vi "AlliGator Compute ROI Decay.vi"(5 "Pixel Threshold High":dbl, 6 "Loop ID":i32, 7 "Pixel Threshold Low":dbl, 8 "error in (no error)":errorcluster, 9 "Decay Peak  Constraints":T2, 10 "ROI Descriptor":T1 {"Contours"."Type" items=["No Selection", "Point", "Line", "Rectangle", "Oval", "Polygon", "Freehand Region", "Annulus", "Unused2", "Unused3", "Broken Line", "Freehand Line", "Rotated Rectangle"]}, 11 "Images":cluster{"Image Sum":T3, "Image Array":T3[]}) -> (0 "error out":errorcluster, 1 "# Valid Pixels":i32, 2 "ROI Center":cluster{"X":i32, "Y":i32}, 3 "Decay Points":dbl[](array[numeric]), 4 "# Pixels":i32)   [LabVIEW 2021, in "AlliGator Decay Processing.lvlib"]
doc: "Extracts the ROI pixel intensities for the different gate images, rejecting pixels not satisfying the intensity-based or peak-intensity based criteria.\n\nA different (faster) approach is used for single-pixel ROIs."
uses:
  AlliGator Decay Processing.lvlib
  <vilib>/vision/Image Controls.llb/IMAQ Image.ctl
  Comparison/Is Valid Number (SGL Array).vi
  Arrays/Replace NaN by 0 (2D SGL).vi/df975b44-f6c5-4554-af30-980613d33749.vi
  Comparison/Is a Valid Number (SGL).vi
  <vilib>/Utility/error.llb/Error Cluster From Error Code.vi
  <vilib>/vision/EDVR.llb/IMAQ ImageToEDVR 2D U8.vi
  <vilib>/vision/EDVR.llb/IMAQ ImageToEDVR 2D I16.vi
  <vilib>/vision/EDVR.llb/IMAQ ImageToEDVR 2D SGL.vi
  <vilib>/vision/EDVR.llb/IMAQ ImageToEDVR 2D U16.vi
  <vilib>/ErrorRing/Error Ring.xnode
  Source Image/AlliGator Source Image.lvlib
  <vilib>/vision/NI_Vision_Development_Module.lvlib
  Arrays/Arrays.lvlib
  Image/Image.lvlib
  Comparison/Comparison.lvlib
  Error/Error.lvlib
  Time/Time.lvlib
panel:
  out "CPU (s)":dbl
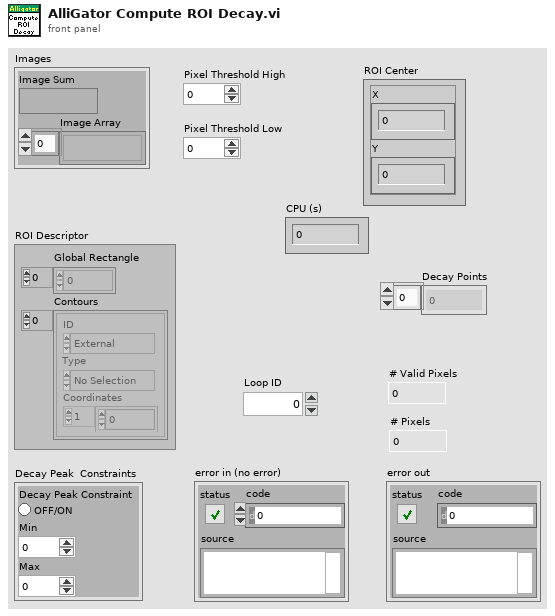
[diagram p1: front panel]
types:
  T1 = typedef "ROI Descriptor" = cluster{"Global Rectangle":i32[], "Contours":cluster{"ID":enum32{"External", "Internal"}, "Type":u32, "Coordinates":i32[]}[]}
  T2 = cluster{"Decay Peak Constraint":bool, "Min":dbl, "Max":dbl}
  T3 = typedef "IMAQ Image.ctl" = refnum<image>
  T4 = typedef "IMAQ Point" = cluster{"X":sgl, "Y":sgl}
  T5 = typedef "Image Type" = u32
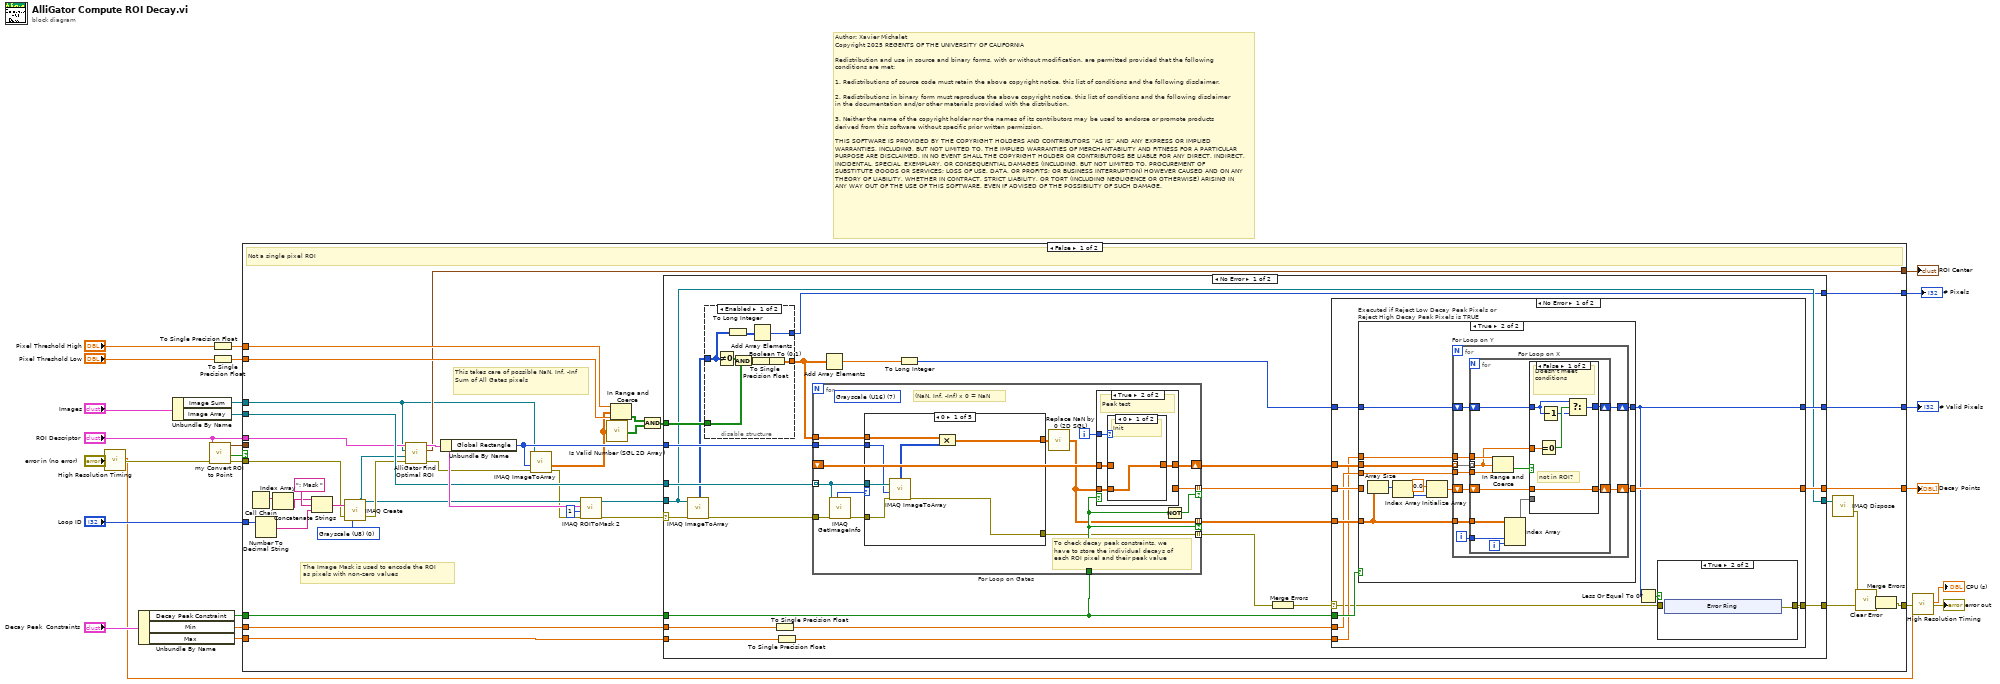
[diagram p0: block diagram]
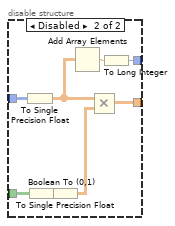
[diagram p2: hidden frame]
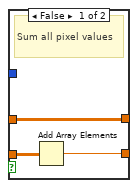
[diagram p3: hidden frame]
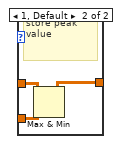
[diagram p4: hidden frame]
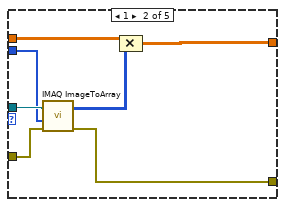
[diagram p5: hidden frame]
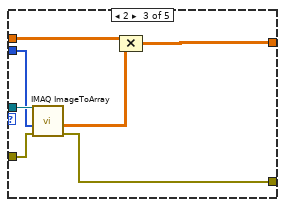
[diagram p6: hidden frame]
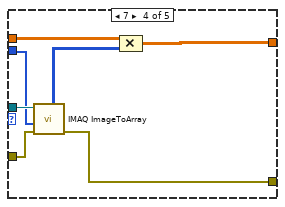
[diagram p7: hidden frame]
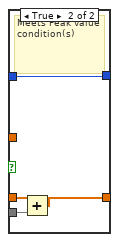
[diagram p11: hidden frame]
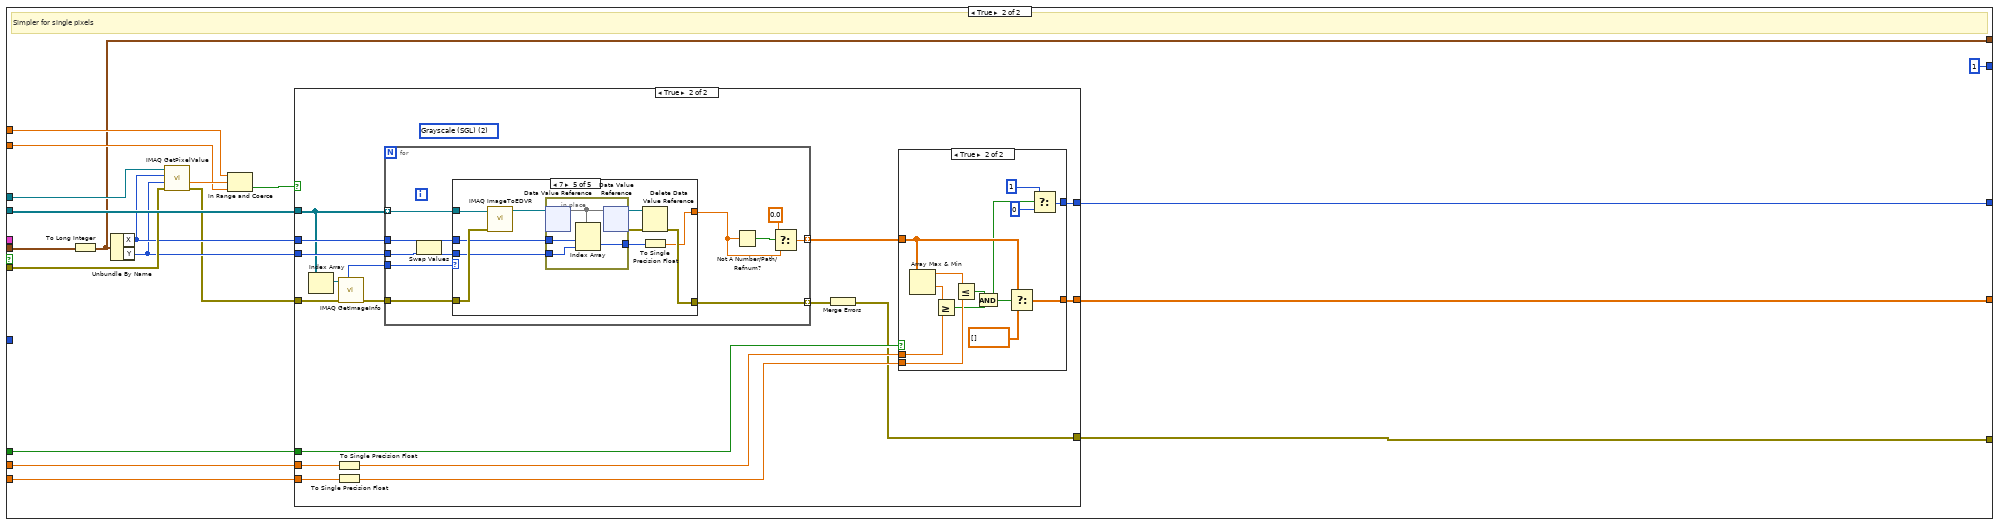
[diagram p14: hidden frame]
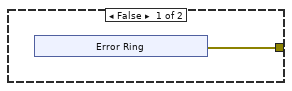
[diagram p15: hidden frame]
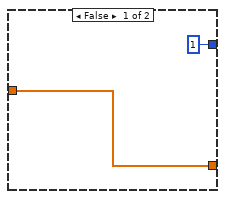
[diagram p16: hidden frame]
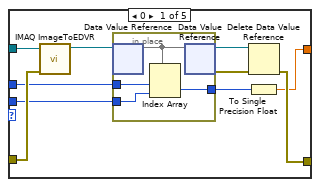
[diagram p17: hidden frame]
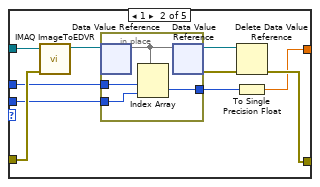
[diagram p18: hidden frame]
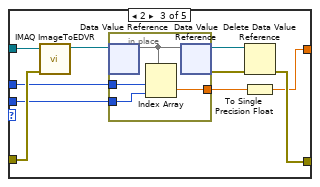
[diagram p19: hidden frame]
diagram:
  # "Author: Xavier Michalet\nCopyright 2025 REGENTS OF THE UNIVERSITY OF CALIFORNIA\n\nRedistribution and use in source and binary forms, with or without modification, are permitted provided that the following conditions are met:\n\n1. Redistributions of source code must retain the above copyright notice, this list of conditions and the following disclaimer.\n\n2. Redistributions in binary form must reproduce the above copyright notice, this list of conditions and the following disclaimer in the documentation and/or other materials provided with the distribution.\n\n3. Neither the name of the copyright holder nor the names of its contributors may be used to endorse or promote products derived from this software without specific prior written permission.\n\nTHIS SOFTWARE IS PROVIDED BY THE COPYRIGHT HOLDERS AND CONTRIBUTORS “AS IS” AND ANY EXPRESS OR IMPLIED WARRANTIES, INCLUDING, BUT NOT LIMITED TO, THE IMPLIED WARRANTIES OF MERCHANTABILITY AND FITNESS FOR A PARTICULAR PURPOSE ARE DISCLAIMED. IN NO EVENT SHALL THE COPYRIGHT HOLDER OR CONTRIBUTORS BE LIABLE FOR ANY DIRECT, INDIRECT, INCIDENTAL, SPECIAL, EXEMPLARY, OR CONSEQUENTIAL DAMAGES (INCLUDING, BUT NOT LIMITED TO, PROCUREMENT OF SUBSTITUTE GOODS OR SERVICES; LOSS OF USE, DATA, OR PROFITS; OR BUSINESS INTERRUPTION) HOWEVER CAUSED AND ON ANY THEORY OF LIABILITY, WHETHER IN CONTRACT, STRICT LIABILITY, OR TORT (INCLUDING NEGLIGENCE OR OTHERWISE) ARISING IN ANY WAY OUT OF THE USE OF THIS SOFTWARE, EVEN IF ADVISED OF THE POSSIBILITY OF SUCH DAMAGE."
  n1 = call "High Resolution Timing.vi"("Error In"="error in (no error)") -> ("elapsed (relative) seconds"=w1:dbl, "Error Out"=w4:errorcluster)  [unwired: 16 in, 1 out]
  n2 = Unbundle By Name("Decay Peak  Constraints") -> ("Decay Peak Constraint"=w23:bool, "Min"=w24:dbl, "Max"=w25:dbl)
  n3 = Unbundle By Name("Images") -> ("Image Sum"=w21:T3, "Image Array"=w13:T3[])
  n4 = call "my Convert ROI to Point.vi"("error in (no error)"=w4, "ROI Descriptor"="ROI Descriptor") -> ("error out"=w9:errorcluster, "Is a Point?"=w8:bool, "Point"=w6:T4)  [unwired: 6 in]
  n5 = To Single Precision Float(number="Pixel Threshold High") -> (single precision float=w19:sgl)
  n6 = To Single Precision Float(number="Pixel Threshold Low") -> (single precision float=w16:sgl)
  n7 = case shown="False" w8 {
    tunnel: w25 -> [w64 w232]
    tunnel: w24 -> [w63 w231]
    tunnel: w23 -> [w62 w233]
    tunnel: w21 -> [w30 w242]
    tunnel: [w29 w226] -> w20
    tunnel: w19 -> [w60 w239]
    tunnel: [w59 1] -> w17
    tunnel: w16 -> [w57 w238]
    tunnel: [w53 w227] -> w15
    tunnel: [w52 w230] -> w14
    tunnel: w13 -> [w51 w243]
    tunnel: [w50 w228] -> w12
    tunnel: w9 -> [w45 w241]
    tunnel: "ROI Descriptor" -> [w48 _]
    tunnel: w6 -> [_ w229]
    tunnel: "Loop ID" -> [w38 _]
    frame False {
      w41 = T5 0 items=["Grayscale (U8)", "Grayscale (I16)", "Grayscale (SGL)", "Complex (CSG)", "RGB (U32)", "HSL (U32)", "RGB (U64)", "Grayscale (U16)"] ("Image Type")
      # "This takes care of possible NaN, Inf, -Inf Sum of All Gates pixels"
      # "The Image Mask is used to encode the ROI\nas pixels with non-zero values"
      # "Not a single pixel ROI"
      n8 = Call Chain() -> (call chain=w39:string[])
      n9 = Number To Decimal String(number=w38) -> (decimal integer string=w37:string)  [unwired: 1 in]
      n10 = Index Array(array=w39) -> (element=w40:string)  [unwired: 1 in]
      n11 = Concatenate Strings(w40, ": Mask " ("string"), w37) -> (w47:string)
      n12 = call "IMAQ Create"("Image Name"=w47, "Image Type"=w41, "error in (no error)"=w45) -> ("New Image"=w42:T3, "error out"=w44:errorcluster)  [unwired: 2 in]
      n13 = call "AlliGator Find Optimal ROI.vi"("error in (no error)"=w44, "ROI Mask"=w42, "Image Sum"=w30, "ROI Descriptor in"=w48) -> ("error out"=w36:errorcluster, "ROI Center"=w50:cluster{"X":i32, "Y":i32}, "ROI Descriptor out"=w55:T1)  [unwired: 5 in]
      n14 = Unbundle By Name(w55) -> ("Global Rectangle"=w35:i32[])
      n15 = call "IMAQ ImageToArray"("error in (no error)"=w36, "Optional Rectangle"=w35, "Image"=w30) -> ("Image Pixels (Float)"=w34:sgl[][], "error out"=w31:errorcluster)  [unwired: 1 in, 3 out]
      n16 = call "IMAQ ROIToMask 2"("error in (no error)"=w31, "Filling Value (255)"=1, "ROI Descriptor"=w55, "Image"=w42) -> ("error out"=w49:errorcluster, "Image Out"=w54:T3)  [unwired: 5 in, 1 out]
      n17 = call "Is Valid Number (SGL 2D Array).vi"("SGL 2D Array"=w34) -> ("Is Valid Number? (2D)"=w32:bool[][])  [unwired: 8 in]
      n18 = In Range and Coerce(upper limit=w60, x=w34, lower limit=w57) -> (In Range?=w33:bool[][])  [unwired: 1 out]
      n19 = Compound Arithmetic op=AND(w33, w32) -> (w58:bool[][])
      n20 = case shown="No Error" w49 {
        selector: w49 -> [w74 w224]
        tunnel: w64 -> [w88 _]
        tunnel: w63 -> [w87 _]
        tunnel: w62 -> [w86 _]
        tunnel: [w71 w224] -> w61
        tunnel: [w65 _] -> w59
        tunnel: w58 -> [w84 _]
        tunnel: w35 -> [w83 _]
        tunnel: w54 -> [w72 w223]
        tunnel: [w81 _] -> w53
        tunnel: [w80 _] -> w52
        tunnel: w51 -> [w77 _]
        tunnel: [w72 w223] -> w43
        frame No Error {
          n21 = call "IMAQ ImageToArray"("error in (no error)"=w74, "Image"=w72) -> ("error out"=w67:errorcluster, "Image Pixels (U8)"=w69:u8[][])  [unwired: 2 in, 3 out]
          n22 = disable-structure shown="Enabled" {
            disable-tunnel: w84 -> [w96 w104]
            disable-tunnel: w69 -> [w91 w102]
            disable-tunnel: [w92 w98] -> w68
            disable-tunnel: [w89 w97] -> w65
            frame Enabled {
              n23 = Not Equal To 0?(x=w91) -> (x != 0?=w95:bool[][])
              n24 = To Long Integer(number=w91) -> (32bit integer=w90:i32[][])
              n25 = And(x=w96, y=w95) -> (x .and. y?=w94:bool[][])
              n26 = Boolean To (0,1)(Boolean=w94) -> (0, 1=w93:i16[][])
              n27 = Add Array Elements(numeric array=w90) -> (sum=w89:i32)
              n28 = To Single Precision Float(number=w93) -> (single precision float=w92:sgl[][])
            }
            frame Disabled {
              n29 = To Single Precision Float(number=w102) -> (single precision float=w100:sgl[][])
              n30 = Boolean To (0,1)(Boolean=w104) -> (0, 1=w103:i16[][])
              n31 = To Single Precision Float(number=w103) -> (single precision float=w99:sgl[][])
              n32 = Add Array Elements(numeric array=w100) -> (sum=w101:sgl)
              n33 = Multiply(x=w100, y=w99) -> (x*y=w98:sgl[][])
              n34 = To Long Integer(number=w101) -> (32bit integer=w97:i32)
            }
          }
          n35 = To Single Precision Float(number=w87) -> (single precision float=w76:sgl)
          n36 = To Single Precision Float(number=w88) -> (single precision float=w75:sgl)
          n37 = for "For Loop on Gates" {
            tunnel: w77 -> [w111] mode=indexing
            tunnel: [w117] -> w79 mode=indexing if=w115
            shift-right: [w119] -> w82
            shift-left: _ -> [w118]
            tunnel: w86 -> [w116]
            tunnel: [w105] -> w78 mode=indexing if=w116
            tunnel: w83 -> [w114]
            tunnel: w68 -> [w112]
            tunnel: [w109] -> w70 mode=indexing
            tunnel: w67 -> [w108]
            i -> [w113]
            (unwired) T5 7 items=["Grayscale (U8)", "Grayscale (I16)", "Grayscale (SGL)", "Complex (CSG)", "RGB (U32)", "HSL (U32)", "RGB (U64)", "Grayscale (U16)"] ("Image Type")
            # "(NaN, Inf, -Inf) x 0 = NaN"
            # "To check decay peak constraints, we have to store the individual decays of each ROI pixel and their peak value"
            n38 = call "IMAQ GetImageInfo"("error in (no error)"=w108, "Image"=w111) -> ("error out"=w106:errorcluster, "Image Type"=w110:T5)  [unwired: 2 in, 6 out]
            n39 = case shown="0" w110 {
              tunnel: [w137 w144 w151 w158 _] -> w107
              tunnel: w114 -> [w132 w138 w145 w152 _]
              tunnel: w112 -> [w136 w143 w150 w157 _]
              tunnel: w111 -> [w135 w142 w149 w156 _]
              tunnel: [w131 w140 w147 w154 w159] -> w109
              tunnel: w106 -> [w134 w141 w148 w155 w159]
              frame 0 {
                n40 = call "IMAQ ImageToArray"("error in (no error)"=w134, "Optional Rectangle"=w132, "Image"=w135) -> ("error out"=w131:errorcluster, "Image Pixels (U8)"=w133:u8[][])  [unwired: 1 in, 3 out]
                n41 = Compound Arithmetic op=MULTIPLY(w136, w133) -> (w137:sgl[][])
              }
              frame 1 {
                n42 = call "IMAQ ImageToArray"("error in (no error)"=w141, "Optional Rectangle"=w138, "Image"=w142) -> ("error out"=w140:errorcluster, "Image Pixels (I16)"=w139:i16[][])  [unwired: 1 in, 3 out]
                n43 = Compound Arithmetic op=MULTIPLY(w143, w139) -> (w144:sgl[][])
              }
              frame 2 {
                n44 = call "IMAQ ImageToArray"("error in (no error)"=w148, "Optional Rectangle"=w145, "Image"=w149) -> ("Image Pixels (Float)"=w146:sgl[][], "error out"=w147:errorcluster)  [unwired: 1 in, 3 out]
                n45 = Compound Arithmetic op=MULTIPLY(w150, w146) -> (w151:sgl[][])
              }
              frame 7 {
                n46 = call "IMAQ ImageToArray"("error in (no error)"=w155, "Optional Rectangle"=w152, "Image"=w156) -> ("Image Pixels (U16)"=w153:u16[][], "error out"=w154:errorcluster)  [unwired: 1 in, 3 out]
                n47 = Compound Arithmetic op=MULTIPLY(w157, w153) -> (w158:sgl[][])
              }
              frame 3, Default {
              }
            }
            n48 = call "Replace NaN by 0 (2D SGL).vi"("Array in"=w107) -> ("Array out"=w105:sgl[][])  [unwired: 8 in]
            n49 = case shown="True" w116 {
              tunnel: w113 -> [_ w126]
              tunnel: w105 -> [w121 w125]
              tunnel: [w122 w124] -> w119
              tunnel: w118 -> [w122 w123]
              tunnel: [w120 _] -> w117
              frame False {
                # "Sum all pixel values"
                n50 = Add Array Elements(numeric array=w121) -> (sum=w120:sgl)
              }
              frame True {
                # "Peak test"
                n51 = case shown="0" w126 {
                  tunnel: w125 -> [w127 w129]
                  tunnel: [w127 w128] -> w124
                  tunnel: w123 -> [_ w130]
                  frame 0 {
                    # "Init"
                  }
                  frame 1, Default {
                    # "store peak value"
                    n52 = Max & Min(x=w130, y=w129) -> (max(x,y)=w128:sgl[][])  [unwired: 1 out]
                  }
                }
              }
            }
            n53 = Not(x=w116) -> (.not. x?=w115:bool)
          }
          n54 = Add Array Elements(numeric array=w68) -> (sum=w85:sgl)
          n55 = To Long Integer(number=w85) -> (32bit integer=w66:i32)
          n56 = Merge Errors(w70) -> (w73:errorcluster)
          n57 = case shown="No Error" w73 {
            selector: w73 -> [w161 w222]
            tunnel: w86 -> [w171 _]
            tunnel: w66 -> [w170 _]
            tunnel: w82 -> [w169 _]
            tunnel: [w163 _] -> w81
            tunnel: [w168 _] -> w80
            tunnel: w79 -> [w167 _]
            tunnel: w78 -> [w166 _]
            tunnel: w76 -> [w165 _]
            tunnel: w75 -> [w164 _]
            tunnel: [w160 w222] -> w71
            frame No Error {
              n58 = case "Executed if Reject Low Decay Peak Pixels or Reject High Decay Peak Pixels is TRUE" shown="True" w171 {
                tunnel: w166 -> [_ w189]
                tunnel: w167 -> [w179 _]
                tunnel: [w179 w182] -> w168
                tunnel: w170 -> [w178 w184]
                tunnel: [w178 w183] -> w163
                tunnel: w169 -> [_ w190]
                tunnel: w165 -> [_ w181]
                tunnel: w164 -> [_ w180]
                frame False {
                }
                frame True {
                  n59 = Array Size(array=w189) -> (size(s)=w188:i32[])
                  n60 = Index Array(array=w188) -> (element=w187:i32)  [unwired: 1 in]
                  n61 = Initialize Array(sgl 0.0 ("element"), w187) -> (w185:sgl[])
                  n62 = for "For Loop on Y" {
                    tunnel: w190 -> [w199] mode=indexing
                    tunnel: w189 -> [w197]
                    tunnel: w181 -> [w198]
                    shift-right: [w192] -> w182
                    shift-left: w185 -> [w193]
                    shift-right: [w194] -> w183
                    shift-left: w184 -> [w195]
                    tunnel: w180 -> [w191]
                    i -> [w196]
                    n63 = for "For Loop on X" {
                      tunnel: w199 -> [w200] mode=indexing
                      tunnel: w198 -> [w202]
                      tunnel: w197 -> [w211]
                      tunnel: w196 -> [w209]
                      shift-right: [w204] -> w194
                      shift-left: w195 -> [w205]
                      shift-right: [w206] -> w192
                      shift-left: w193 -> [w208]
                      tunnel: w191 -> [w203]
                      i -> [w210]
                      n64 = In Range and Coerce(upper limit=w203, x=w200, lower limit=w202) -> (In Range?=w201:bool)  [unwired: 1 out]
                      n65 = Index Array(array=w211, index (dim 1)=w209, index (dim 2)=w210) -> (element=w207:sgl[])  [unwired: 1 in]
                      n66 = case shown="False" w201 {
                        tunnel: w208 -> [w217 w221]
                        tunnel: w207 -> [_ w220]
                        tunnel: [w217 w219] -> w206
                        tunnel: w205 -> [w213 w218]
                        tunnel: w200 -> [w216 _]
                        tunnel: [w214 w218] -> w204
                        frame False {
                          # "not in ROI?"
                          # "Doesn't meet conditions"
                          n67 = Equal To 0?(x=w216) -> (x = 0?=w215:bool)
                          n68 = Decrement(x=w213) -> (x-1=w212:i32)
                          n69 = Select(t=w213, s=w215, f=w212) -> (s? t:f=w214:i32)
                        }
                        frame True {
                          # "Meets Peak value condition(s)"
                          n70 = Add(x=w221, y=w220) -> (x+y=w219:sgl[])
                        }
                      }
                    }
                  }
                }
              }
              n71 = Less Or Equal To 0?(x=w163) -> (x <= 0?=w162:bool)
              n72 = case shown="True" w162 {
                tunnel: w161 -> [w172 _]
                tunnel: [w172 w173] -> w160
                frame False {
                }
                frame True {
                  n73 = xnode "Error Ring"() -> ("error out"=w173:errorcluster)
                }
              }
            }
            frame Error {
            }
          }
        }
        frame Error {
        }
      }
      n74 = call "IMAQ Dispose"("Image"=w43) -> ("error out"=w28:errorcluster)  [unwired: 5 in]
      n75 = call "Clear Error.vi"("Error In"=w28) -> ("no Error Out"=w27:errorcluster)  [unwired: 8 in]
      n76 = Merge Errors(w27, w61) -> (w29:errorcluster)
    }
    frame True {
      # "Simpler for single pixels"
      n77 = To Long Integer(number=w229) -> (32bit integer=w228:cluster{"X":i32, "Y":i32})
      n78 = Unbundle By Name(w228) -> ("X"=w236:i32, "Y"=w235:i32)
      n79 = call "IMAQ GetPixelValue"("Image"=w242, "X Coordinate"=w236, "Y Coordinate"=w235, "error in (no error)"=w241) -> ("Pixel Value (Float)"=w240:sgl, "error out"=w234:errorcluster)  [unwired: 2 in, 3 out]
      n80 = In Range and Coerce(upper limit=w239, x=w240, lower limit=w238) -> (In Range?=w237:bool)  [unwired: 1 out]
      n81 = case shown="True" w237 {
        tunnel: w243 -> [_ w250]
        tunnel: w236 -> [_ w265]
        tunnel: w235 -> [_ w264]
        tunnel: w234 -> [_ w253]
        tunnel: w233 -> [_ w263]
        tunnel: w232 -> [_ w261]
        tunnel: w231 -> [_ w260]
        tunnel: [_ w257] -> w230
        tunnel: [_ w254] -> w227
        tunnel: [w244 w255] -> w226
        frame False {
          n82 = xnode "Error Ring"() -> ("error out"=w244:errorcluster)
        }
        frame True {
          (unwired) T5 2 items=["Grayscale (U8)", "Grayscale (I16)", "Grayscale (SGL)", "Complex (CSG)", "RGB (U32)", "HSL (U32)", "RGB (U64)", "Grayscale (U16)"] ("Image Type")
          n83 = Index Array(array=w250) -> (element=w249:T3)  [unwired: 1 in]
          n84 = To Single Precision Float(number=w260) -> (single precision float=w259:sgl)
          n85 = To Single Precision Float(number=w261) -> (single precision float=w258:sgl)
          n86 = call "IMAQ GetImageInfo"("error in (no error)"=w253, "Image"=w249) -> ("error out"=w252:errorcluster, "Image Type"=w251:T5)  [unwired: 2 in, 6 out]
          n87 = for {
            tunnel: w250 -> [w290] mode=indexing
            tunnel: w265 -> [w292]
            tunnel: w264 -> [w291]
            tunnel: w252 -> [w288]
            tunnel: [w284] -> w262 mode=indexing
            tunnel: [w283] -> w256 mode=indexing
            tunnel: w251 -> [w289]
            n88 = Swap Values(12:w292, 14:w291) -> (1:w282:i32, 3:w281:i32)  [unwired: 1 in]
            n89 = case shown="7" w289 {
              tunnel: w290 -> [w302 w316 w330 _ w345]
              tunnel: w288 -> [w298 w312 w326 w335 w342]
              tunnel: w282 -> [w297 w311 w325 _ w341]
              tunnel: w281 -> [w296 w310 w324 _ w340]
              tunnel: [w293 w307 w321 _ w337] -> w285
              tunnel: [w294 w308 w322 w335 w338] -> w283
              frame 0 {
                n90 = call-poly <vilib>:"IMAQ ImageToEDVR.vi"("error in (no error)"=w298, "Image"=w302) -> ("EDVR 2D U8"=w301:refnum<data-value>)  [unwired: 7 in, 2 out]
                n91 = in-place {
                  in-place-border: w297 -> [w305]
                  in-place-border: w296 -> [w304]
                  in-place-border: [w303] -> w295
                  n92 = in-place-dvr #1(w301) -> (w306:u8[][])  [unwired: 1 out]
                  n93 = Index Array(array=w306, index (row)=w305, index (col)=w304) -> (element=w303:u8)
                  n94 = in-place-dvr #1(w306) -> (w300:refnum<data-value>, w299:errorcluster)
                }
                n95 = Delete Data Value Reference(data value reference=w300, error in=w299) -> (error out=w294:errorcluster)  [unwired: 1 out]
                n96 = To Single Precision Float(number=w295) -> (single precision float=w293:sgl)
              }
              frame 1 {
                n97 = call-poly <vilib>:"IMAQ ImageToEDVR.vi"("error in (no error)"=w312, "Image"=w316) -> ("EDVR 2D I16"=w315:refnum<data-value>)  [unwired: 7 in, 2 out]
                n98 = in-place {
                  in-place-border: w311 -> [w319]
                  in-place-border: w310 -> [w318]
                  in-place-border: [w317] -> w309
                  n99 = in-place-dvr #2(w315) -> (w320:i16[][])  [unwired: 1 out]
                  n100 = Index Array(array=w320, index (row)=w319, index (col)=w318) -> (element=w317:i16)
                  n101 = in-place-dvr #2(w320) -> (w314:refnum<data-value>, w313:errorcluster)
                }
                n102 = Delete Data Value Reference(data value reference=w314, error in=w313) -> (error out=w308:errorcluster)  [unwired: 1 out]
                n103 = To Single Precision Float(number=w309) -> (single precision float=w307:sgl)
              }
              frame 2 {
                n104 = call-poly <vilib>:"IMAQ ImageToEDVR.vi"("error in (no error)"=w326, "Image"=w330) -> ("EDVR 2D SGL"=w329:refnum<data-value>)  [unwired: 7 in, 2 out]
                n105 = in-place {
                  in-place-border: w325 -> [w333]
                  in-place-border: w324 -> [w332]
                  in-place-border: [w331] -> w323
                  n106 = in-place-dvr #3(w329) -> (w334:sgl[][])  [unwired: 1 out]
                  n107 = Index Array(array=w334, index (row)=w333, index (col)=w332) -> (element=w331:sgl)
                  n108 = in-place-dvr #3(w334) -> (w328:refnum<data-value>, w327:errorcluster)
                }
                n109 = Delete Data Value Reference(data value reference=w328, error in=w327) -> (error out=w322:errorcluster)  [unwired: 1 out]
                n110 = To Single Precision Float(number=w323) -> (single precision float=w321:sgl)
              }
              frame 3, Default {
              }
              frame 7 {
                n111 = call-poly <vilib>:"IMAQ ImageToEDVR.vi"("error out"=w342, "Image"=w345) -> ("EDVR 2D U16"=w344:refnum<data-value>)  [unwired: 7 in, 2 out]
                n112 = in-place {
                  in-place-border: w341 -> [w348]
                  in-place-border: w340 -> [w347]
                  in-place-border: [w346] -> w339
                  n113 = in-place-dvr #4(w344) -> (w349:u16[][])  [unwired: 1 out]
                  n114 = Index Array(array=w349, index (row)=w348, index (col)=w347) -> (element=w346:u16)
                  n115 = in-place-dvr #4(w349) -> (w336:refnum<data-value>, w343:errorcluster)
                }
                n116 = Delete Data Value Reference(data value reference=w336, error in=w343) -> (error out=w338:errorcluster)  [unwired: 1 out]
                n117 = To Single Precision Float(number=w339) -> (single precision float=w337:sgl)
              }
            }
            n118 = Not A Number/Path/Refnum?(number/path/refnum=w285) -> (NaN/Path/Refnum?=w287:bool)
            n119 = Select(t=sgl 0.0, s=w287, f=w285) -> (s? t:f=w284:sgl)
          }
          n120 = Merge Errors(w256) -> (w255:errorcluster)
          n121 = case shown="True" w263 {
            tunnel: w262 -> [w267 w274]
            tunnel: [w267 w272] -> w257
            tunnel: w258 -> [_ w279]
            tunnel: w259 -> [_ w277]
            tunnel: [1 ("f") w269] -> w254
            frame False {
            }
            frame True {
              n122 = Array Max & Min(array=w274) -> (max value=w280:sgl, min value=w278:sgl)  [unwired: 2 out]
              n123 = Greater Or Equal?(x=w278, y=w277) -> (x >= y?=w276:bool)
              n124 = Less Or Equal?(x=w280, y=w279) -> (x <= y?=w275:bool)
              n125 = And(x=w275, y=w276) -> (x .and. y?=w270:bool)
              n126 = Select(t=w274, s=w270, f=sgl[] []) -> (s? t:f=w272:sgl[])
              n127 = Select(t=1 ("Numeric"), s=w270, f=0) -> (s? t:f=w269:i32)
            }
          }
        }
      }
    }
  }
  "ROI Center" <- w12
  "# Pixels" <- w17
  "# Valid Pixels" <- w15
  "Decay Points" <- w14
  n128 = call "High Resolution Timing.vi"("relative seconds (NaN)"=w1, "Error In"=w20) -> ("elapsed (relative) seconds"=→"CPU (s)":dbl, "Error Out"=→"error out":errorcluster)  [unwired: 15 in, 1 out]
